vi "1.2 Producer Consumer Test3.vi"() -> ()   [LabVIEW 2018]
uses:
  <vilib>/DAQmx/read.llb/DAQmx Read (Analog DBL 1Chan 1Samp).vi
  <vilib>/DAQmx/miscellaneous.llb/DAQmx Fill In Error Info.vi
  <vilib>/DAQmx/configure/timing.llb/DAQmx Timing (Sample Clock).vi
  <vilib>/DAQmx/create/channels.llb/DAQmx Create Channel (AI-Voltage-Basic).vi
panel:
  out "Waveform Chart 2":dbl(graph)
  out "Numeric 2":dbl
  in  "stop 2":bool
  out "Numeric":dbl
  out "Waveform Chart":dbl(graph)
  in  "stop":bool
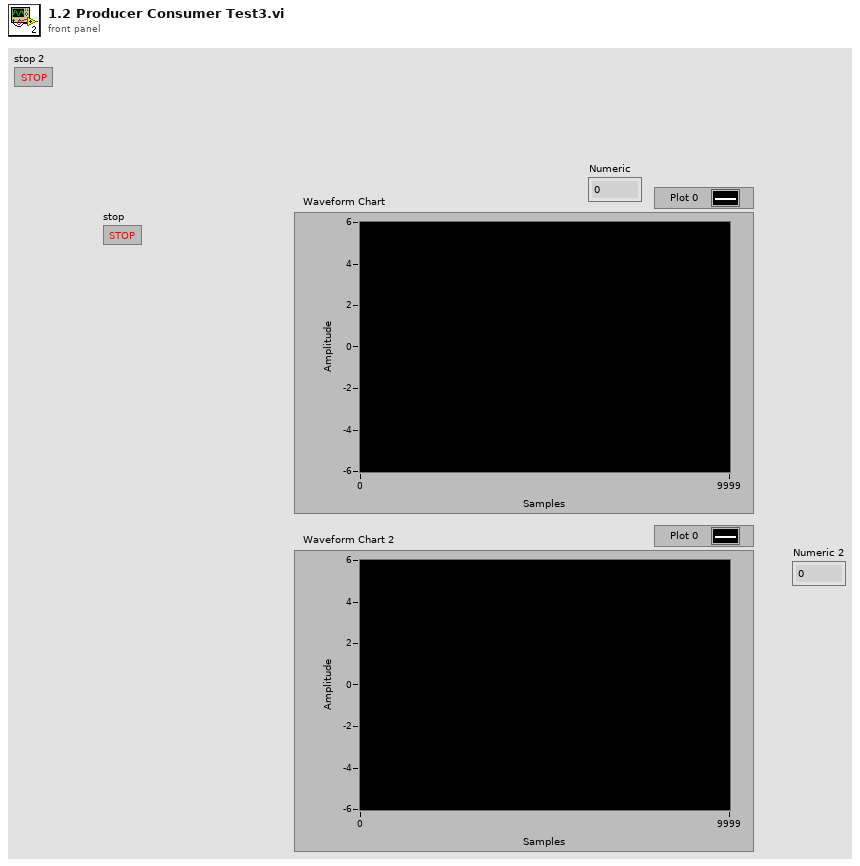
[diagram p1: front panel]
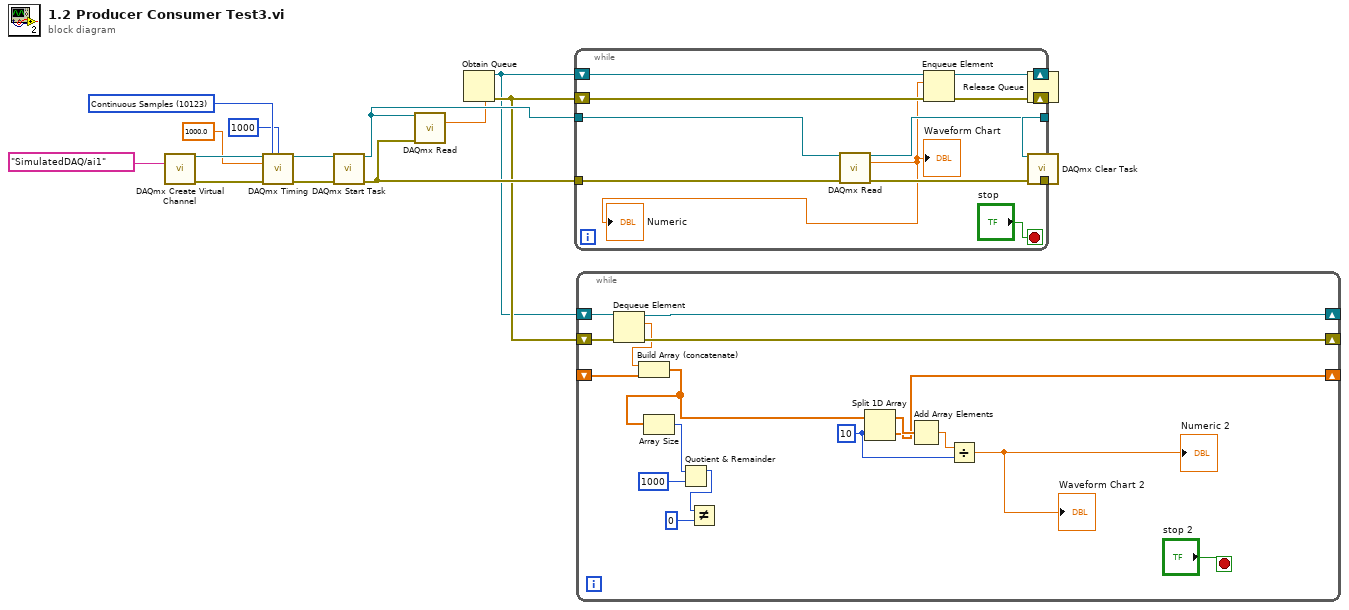
[diagram p0: block diagram]
diagram:
  w13 = 10123 items=["Finite Samples"=10178, "Continuous Samples"=10123, "Hardware Timed Single Point"=12522] ("sample mode")
  n1 = call-poly <vilib>:"DAQmx Create Virtual Channel.vi"("physical channels"=tag "SimulatedDAQ/ai1") -> ("task out"=w14:refnum<k21>, "error out"=w15:errorcluster)  [unwired: 13 in]
  n2 = call-poly <vilib>:"DAQmx Timing.vi"("task/channels in"=w14, "sample mode"=w13, "samples per channel"=1000, "rate"=1000.0, "error in"=w15) -> ("task out"=w16:refnum<k21>, "error out"=w17:errorcluster)  [unwired: 9 in]
  n3 = call <vilib>:"DAQmx Start Task.vi"("task/channels in"=w16, "error in"=w17) -> ("task out"=w5:refnum<k21>, "error out"=w6:errorcluster)  [unwired: 12 in]
  n4 = call-poly <vilib>:"DAQmx Read.vi"("task/channels in"=w5, "error in"=w6) -> ("data"=w4:dbl)  [unwired: 11 in, 2 out]
  n5 = Obtain Queue(element data type=w4) -> (queue out=w1:refnum<queue>, error out=w3:errorcluster)  [unwired: 4 in, 1 out]
  n6 = while {
    tunnel: w6 -> [w27]
    tunnel: [w26] -> w11
    tunnel: [w25] -> w10
    shift-right: [w22] -> w8
    shift-left: w1 -> [w24]
    shift-right: [w21] -> w7
    shift-left: w3 -> [w23]
    tunnel: w5 -> [w19]
    stop <- "stop" stop-if-true
    n7 = call-poly <vilib>:"DAQmx Read.vi"("task/channels in"=w19, "error in"=w27) -> ("task out"=w26:refnum<k21>, "data"=w18:dbl, "error out"=w25:errorcluster)  [unwired: 11 in]
    "Waveform Chart" <- w18
    "Numeric" <- w18
    n8 = Enqueue Element(queue=w24, element=w18, error in (no error)=w23) -> (queue out=w22:refnum<queue>, error out=w21:errorcluster)  [unwired: 1 in, 1 out]
  }
  n9 = while {
    shift-right: [w42] -> _
    shift-left: w1 -> [w44]
    shift-right: [w41] -> _
    shift-left: w3 -> [w43]
    shift-right: [w29] -> _
    shift-left: _ -> [w28]
    stop <- "stop 2" stop-if-true
    w32 = 10 ("index")
    n10 = Dequeue Element(queue=w44, error in (no error)=w43) -> (queue out=w42:refnum<queue>, element=w39:dbl, error out=w41:errorcluster)  [unwired: 1 in, 1 out]
    n11 = Build Array (concatenate)(w39, w28) -> (w34:dbl[])
    n12 = Array Size(array=w34) -> (size(s)=w38:i32)
    n13 = Quotient & Remainder(x=w38, y=1000) -> (x-y*floor(x/y)=w36:i32)  [unwired: 1 out]
    n14 = Not Equal?(x=w36, y=0) -> ()  [unwired: 1 out]
    n15 = Split 1D Array(array=w34, index=w32) -> (first subarray=w30:dbl[], second subarray=w29:dbl[])
    n16 = Add Array Elements(numeric array=w30) -> (sum=w33:dbl)
    n17 = Divide(x=w33, y=w32) -> (x/y=→"Numeric 2" →"Waveform Chart 2":dbl)
  }
  n18 = Release Queue(queue=w8, error in (no error)=w7) -> ()  [unwired: 1 in, 3 out]
  n19 = call <vilib>:"DAQmx Clear Task.vi"("task in"=w11, "error in"=w10) -> ()  [unwired: 13 in, 1 out]
